vi "VNA.vi"() -> ()   [LabVIEW 2022 SP3]
uses:
  C:/Users/Public/OneDrive/Desktop/Control 1.ctl
  <vilib>/Utility/file.llb/Write Delimited Spreadsheet (DBL).vi
  Agilent ENA Series/Agilent ENA Series.lvlib
panel:
  in  "Average":i32=1
  in  "wait time (ms)":dbl=15000.0
  in  "Smoothing State (F: Off)":bool
  in  "IF Bandwidth (100000.0)":dbl=1000.0 format="%^.1e"
  in  "Average Factor (16)":i32=16
  in  "Averaging State (F: Off)":bool
  in  "Continuous Sweep (T: Enable)":bool=TRUE
  in  "Point Trigger (F: Disable)":bool
  in  "Trigger Source":u16(ring) items=["Internal", "External", "Manual", "BUS"]
  in  "Stop (MHz)":dbl format="%^.2e"
  in  "Start (Mhz)":dbl=1.0 format="%^.2e"
  in  "Number of Measurement Points":i32=1001
  in  "Power Level (dBm)":dbl=-5.0 format="%^.2g"
  in  "file path (dialog if empty)":path=path "D:/LabData/XiaoWang_Group_data_2024on/Fan Fei/NOEMS/1-10-2024/7.txt"
  in  "Measurement Parameters":u16(ring)=1 items=["S11", "S21", "S31", "S41", "S12", "S22", "S32", "S42", "S13", "S23", "S33", "S43", "S14", "S24", "S34", "S44", "A", "B", "C", "D", "R1", "R2", "R3", "R4"]
  out "Waveform Graph":T1
  in  "Safe Mode Maximum Power Level (30)":dbl=30.0
  in  "Safe Mode Minimum Power Level (-200)":dbl=-200.0
  in  "Tolerance Level (5)":dbl=5.0
  in  "Power Level Offset (0)":dbl
  in  "Port ( 1)":i32=1
  in  "Channel (1)":i32=1
  in  "Enable Safe Mode (T: Enabled)":bool=TRUE
  in  "Enable Receiver Leveling (T: Enabled)":bool=TRUE
  in  "Reset? (T: Yes)":bool=TRUE
  in  "ID Query? (T: Yes)":bool=TRUE
  in  "VISA resource name":refnum<visa-resource-name>="GPIB0::27::INSTR"
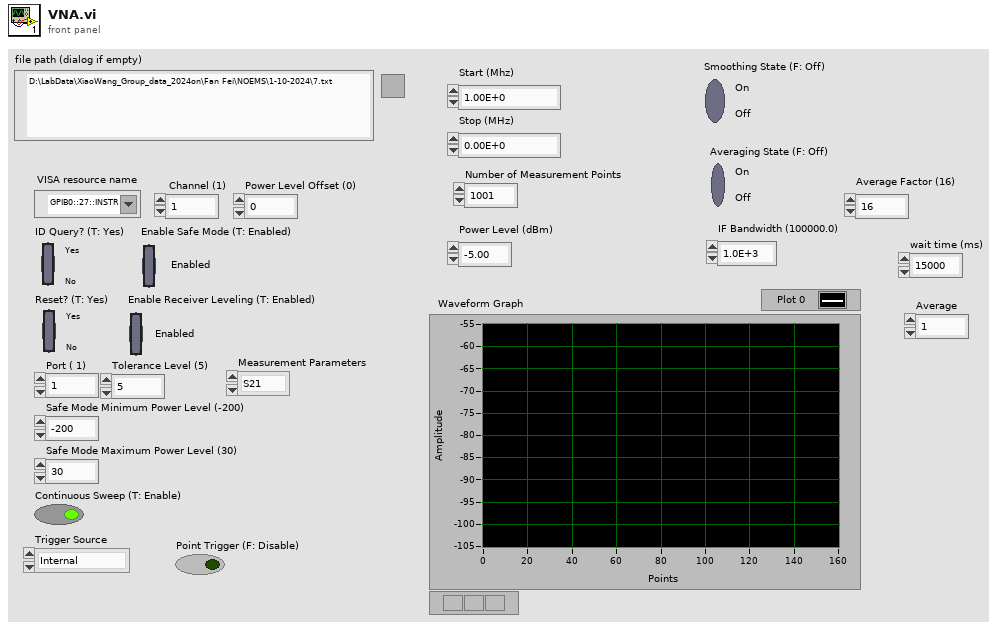
[diagram p1: front panel]
types:
  T1 = typedef "Control 1.ctl" = dbl[]
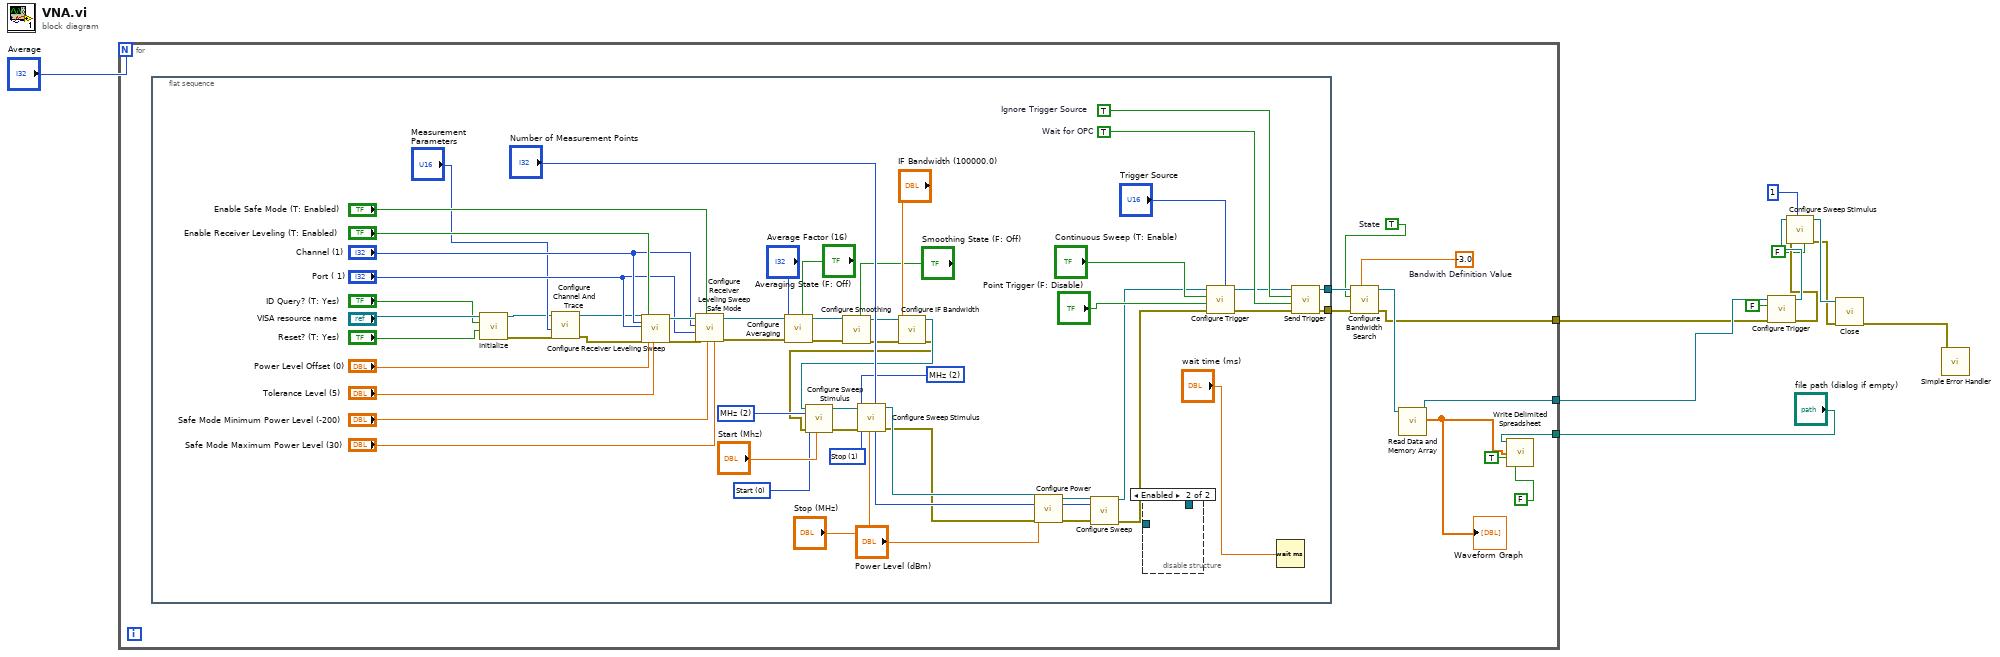
[diagram p0: block diagram]
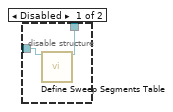
[diagram p2: hidden frame]
diagram:
  n1 = for {
    N: "Average" -> [_]
    tunnel: [w23] -> w11
    tunnel: [w17] -> w9
    tunnel: "file path (dialog if empty)" -> [w15]
    w19 = TRUE  # State
    w20 = -3.0  # Bandwith Definition Value
    n2 = flat-sequence {
      tunnel: [w77] -> w21
      tunnel: [w25] -> w18
      frame #0 {
        w52 = u16 2 items=["Hz", "kHz", "MHz", "GHz", "dBm", "s", "V"] ("Unit (0: Hz)")
        w53 = u16 2 items=["Hz", "kHz", "MHz", "GHz", "dBm", "s", "V"] ("Unit (0: Hz)")
        w54 = u16 1 items=["Start", "Stop", "Center", "Span"] ("Stimulus (0: Start)")
        w55 = u16 0 items=["Start", "Stop", "Center", "Span"] ("Stimulus (0: Start)")
        w78 = TRUE  # Wait for OPC
        w79 = TRUE  # Ignore Trigger Source
        n3 = call "Initialize.vi"("Reset? (T: Yes)"="Reset? (T: Yes)", "ID Query? (T: Yes)"="ID Query? (T: Yes)", "VISA resource name"="VISA resource name") -> ("error out"=w37:errorcluster, "VISA resource name out"=w41:refnum<visa-resource-name>)  [unwired: 7 in]
        n4 = call "Configure Channel And Trace.vi"("error in (no error)"=w37, "Measurement Parameters (0: S11)"="Measurement Parameters", "VISA resource name"=w41) -> ("error out"=w36:errorcluster, "VISA resource name out"=w40:refnum<visa-resource-name>)  [unwired: 7 in]
        n5 = call "Configure Receiver Leveling Sweep.vi"("VISA resource name"=w40, "Channel (1)"="Channel (1)", "Port ( 1)"="Port ( 1)", "error in (no error)"=w36, "Enable Receiver Leveling (F: Disabled)"="Enable Receiver Leveling (T: Enabled)", "Power Level Offset (0)"="Power Level Offset (0)", "Tolerance Level (5)"="Tolerance Level (5)") -> ("VISA resource name out"=w72:refnum<visa-resource-name>, "error out"=w35:errorcluster)  [unwired: 11 in]
        n6 = call "Configure Receiver Leveling Sweep Safe Mode.vi"("Safe Mode Maximum Power Level (30)"="Safe Mode Maximum Power Level (30)", "Safe Mode Minimum Power Level (-200)"="Safe Mode Minimum Power Level (-200)", "Enable Safe Mode (F: Disabled)"="Enable Safe Mode (T: Enabled)", "error in (no error)"=w35, "Port ( 1)"="Port ( 1)", "Channel (1)"="Channel (1)", "VISA resource name"=w72) -> ("error out"=w34:errorcluster, "VISA resource name out"=w39:refnum<visa-resource-name>)  [unwired: 3 in]
        n7 = call "Configure Averaging.vi"("Averaging State (F: Off)"="Averaging State (F: Off)", "error in (no error)"=w34, "Factor (16)"="Average Factor (16)", "VISA resource name"=w39) -> ("error out"=w33:errorcluster, "VISA resource name out"=w48:refnum<visa-resource-name>)  [unwired: 6 in]
        n8 = call "Configure Smoothing.vi"("Smoothing State (F: Off)"="Smoothing State (F: Off)", "error in (no error)"=w33, "VISA resource name"=w48) -> ("error out"=w32:errorcluster, "VISA resource name out"=w47:refnum<visa-resource-name>)  [unwired: 7 in]
        n9 = call "Configure IF Bandwidth.vi"("error in (no error)"=w32, "IF Bandwidth (100000.0)"="IF Bandwidth (100000.0)", "VISA resource name"=w47) -> ("error out"=w31:errorcluster, "VISA resource name out"=w46:refnum<visa-resource-name>)  [unwired: 7 in]
        n10 = call "Configure Sweep Stimulus.vi"("Parameter (0.0)"="Start (Mhz)", "error in (no error)"=w31, "Stimulus (0: Start)"=w55, "Unit (0: Hz)"=w53, "VISA resource name"=w46) -> ("error out"=w30:errorcluster, "VISA resource name out"=w59:refnum<visa-resource-name>)  [unwired: 5 in]
        n11 = call "Configure Sweep Stimulus.vi"("Parameter (0.0)"="Stop (MHz)", "error in (no error)"=w30, "Stimulus (0: Start)"=w54, "Unit (0: Hz)"=w52, "VISA resource name"=w59) -> ("error out"=w29:errorcluster, "VISA resource name out"=w58:refnum<visa-resource-name>)  [unwired: 5 in]
        n12 = call "Configure Power.vi"("VISA resource name"=w58, "Power Level (0.0)"="Power Level (dBm)", "error in (no error)"=w29) -> ("VISA resource name out"=w61:refnum<visa-resource-name>, "error out"=w28:errorcluster)  [unwired: 11 in]
        n13 = call "Configure Sweep.vi"("VISA resource name"=w61, "Number of Measurement Points (201)"="Number of Measurement Points", "error in (no error)"=w28) -> ("VISA resource name out"=w38:refnum<visa-resource-name>, "error out"=w27:errorcluster)  [unwired: 11 in]
        n14 = disable-structure shown="Enabled" {
          disable-tunnel: _ -> [w81 _]
          disable-tunnel: [w80 _] -> _
          frame Disabled {
            n15 = call <instrlib>:"Define Sweep Segments Table.vi"("VISA resource name"=w81) -> ("VISA resource name out"=w80:refnum<visa-resource-name>)  [unwired: 17 in, 1 out]
          }
          frame Enabled {
          }
        }
        n16 = call "Configure Trigger.vi"("Trigger Source (0: Internal)"="Trigger Source", "error in (no error)"=w27, "Point Trigger (F: Disable)"="Point Trigger (F: Disable)", "Continuous Sweep (T: Enable)"="Continuous Sweep (T: Enable)", "VISA resource name"=w38) -> ("error out"=w26:errorcluster, "VISA resource name out"=w73:refnum<visa-resource-name>)  [unwired: 5 in]
        n17 = Wait (ms)(milliseconds to wait="wait time (ms)") -> ()  [unwired: 1 out]
        n18 = call "Send Trigger.vi"("error in (no error)"=w26, "Wait for OPC (F: Do not Wait)"=w78, "Ignore Trigger Source (F: Do not Ignore)"=w79, "VISA resource name"=w73) -> ("error out"=w25:errorcluster, "VISA resource name out"=w77:refnum<visa-resource-name>)  [unwired: 6 in]
      }
    }
    n19 = call "Configure Bandwidth Search.vi"("Bandwidth Definition Value (-3.0)"=w20, "error in (no error)"=w18, "Result Display State (F: Disable)"=w19, "VISA resource name"=w21) -> ("error out"=w17:errorcluster, "VISA resource name out"=w22:refnum<visa-resource-name>)  [unwired: 6 in]
    n20 = call "Read Data and Memory Array.vi"("VISA resource name"=w22) -> ("Primary / Real"=w16:dbl[], "VISA resource name out"=w23:refnum<visa-resource-name>)  [unwired: 7 in, 2 out]
    "Waveform Graph" <- w16
    n21 = call-poly <vilib>:"Write Delimited Spreadsheet.vi"("file path (dialog if empty)"=w15, "1D data"=w16, "append to file? (new file:F)"=TRUE, "transpose? (no:F)"=FALSE) -> ()  [unwired: 10 in, 2 out]
  }
  n22 = call "Configure Trigger.vi"("error in (no error)"=w9, "Continuous Sweep (T: Enable)"=FALSE, "VISA resource name"=w11) -> ("error out"=w6:errorcluster, "VISA resource name out"=w8:refnum<visa-resource-name>)  [unwired: 7 in]
  n23 = call "Configure Sweep Stimulus.vi"("Signal Output (T: On)"=FALSE, "Channel (1)"=1, "error in (no error)"=w6, "VISA resource name"=w8) -> ("error out"=w5:errorcluster, "VISA resource name out"=w7:refnum<visa-resource-name>)  [unwired: 6 in]
  n24 = call "Close.vi"("error in (no error)"=w5, "VISA resource name"=w7) -> ("error out"=w12:errorcluster)  [unwired: 9 in]
  n25 = call <vilib>:"Simple Error Handler.vi"("error in (no error)"=w12) -> ()  [unwired: 4 in, 5 out]
